vi "Contains Mouse.vi"(0 "FSM.Node":refnum<class "FSM.Node.lvclass">, 7 "Coords":T1) -> (8 "contains mouse":bool)   [LabVIEW 2020, in "FSM.Node.lvclass"]
uses:
  FSM.Node.lvclass
  <vilib>/Utility/miscctls.llb/LVPoint32TypeDef.ctl
  FSM.Node.lvclass/FSM.Node.ctl
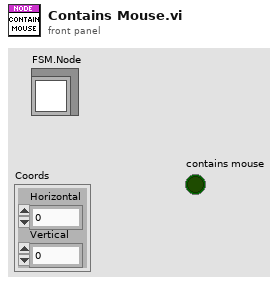
[diagram p1: front panel]
types:
  T1 = typedef "LVPoint32TypeDef.ctl" = cluster{"Horizontal":i32, "Vertical":i32}
  T2 = cluster{"left":i16, "top":i16, "right":i16, "bottom":i16}
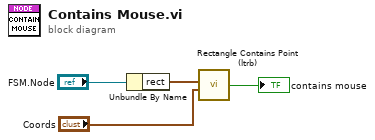
[diagram p0: block diagram]
diagram:
  n1 = Unbundle By Name("FSM.Node") -> ("rect"=w3:T2)
  n2 = call "Rectangle Contains Point (ltrb).vi"("Point"="Coords", "Rectangle"=w3) -> ("Contained?"=→"contains mouse":bool)  [unwired: 4 in]
